vi "Write Prompts.vi"(8 "error in (no error)":errorcluster, 10 "Prompts":bool=TRUE, 11 "Manual PSU in":refnum<class "Manual PSU.lvclass">) -> (0 "error out":errorcluster, 3 "Manual PSU out":refnum<class "Manual PSU.lvclass">)   [LabVIEW 2020, in "Manual PSU.lvclass"]
uses:
  Manual PSU.lvclass
  Manual PSU.lvclass/Manual PSU.ctl
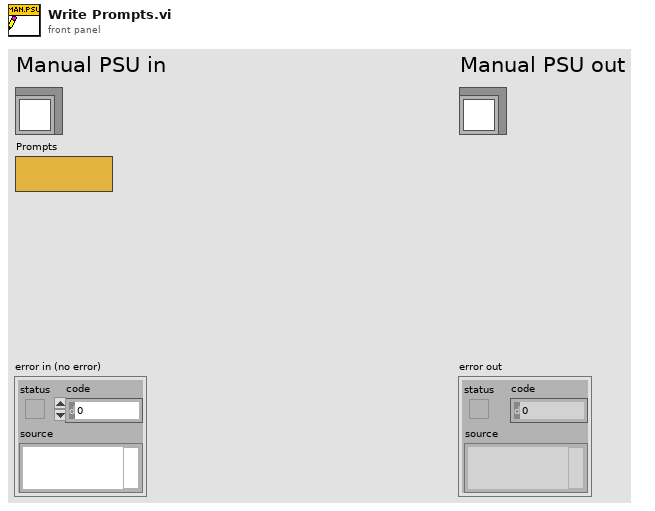
[diagram p1: front panel]
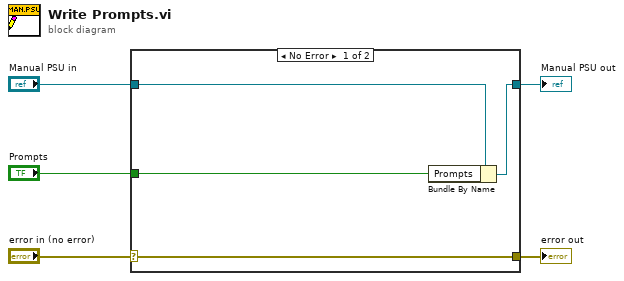
[diagram p0: block diagram]
diagram:
  n1 = case shown="No Error" "error in (no error)" {
    selector: "error in (no error)" -> [w9 w10]
    tunnel: [w9 w10] -> w4
    tunnel: [w7 w11] -> w2
    tunnel: "Manual PSU in" -> [w8 w11]
    tunnel: "Prompts" -> [w6 _]
    frame No Error {
      n2 = Bundle By Name(cluster=w8, "Prompts"=w6) -> (w7:refnum<class "Manual PSU.lvclass">)
    }
    frame Error {
    }
  }
  "error out" <- w4
  "Manual PSU out" <- w2
